vi "mb Convert [U8] to SGL.vi"(2 "Data [ ]":u8[](array[numeric]), 4 "Byte Offset":u16=1) -> (6 "SGL Data [ ]":sgl[](array[numeric]), 7 "SGL Data":sgl)   [LabVIEW 2009]
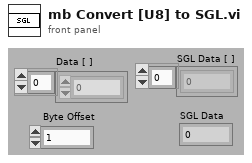
[diagram p1: front panel]
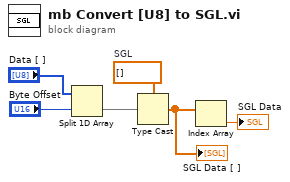
[diagram p0: block diagram]
diagram:
  w2 = sgl[] []  # SGL
  n1 = Split 1D Array(array="Data [ ]", index="Byte Offset") -> (second subarray=w3:u8[])  [unwired: 1 out]
  n2 = Type Cast(type=w2, x=w3) -> (*(type *) &x=w1:sgl[])
  "SGL Data [ ]" <- w1
  n3 = Index Array(array=w1) -> (element=→"SGL Data":sgl)  [unwired: 1 in]
